vi "SetGetMeasMode - Test.vi"() -> ()   [LabVIEW 2017]
uses:
  AT901 API/TypeDefinitions/ES_MeasMode.ctl
panel:
  out "Command 2":string
  out "Respond 2":string[](array[string])
  out "ES_MeasMode 2":T1
  out "Command":string
  out "Respond":string[](array[string])
  in  "ES_MeasMode":T1
  out "error out":errorcluster
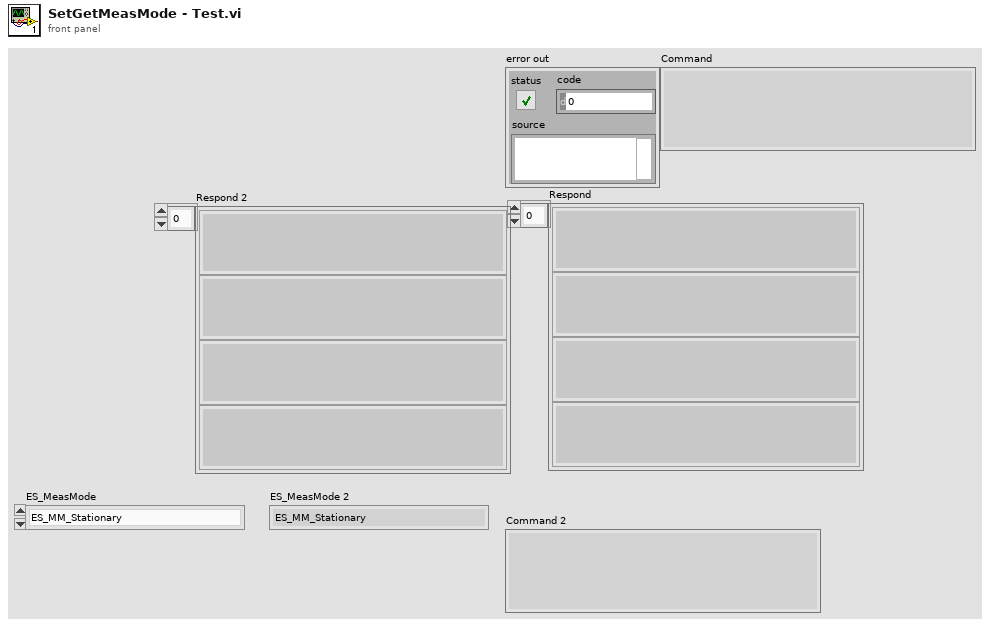
[diagram p1: front panel]
types:
  T1 = typedef "ES_MeasMode.ctl" = enum32{"ES_MM_Stationary", "ES_MM_ContinuousTime", "ES_MM_ContinuousDistance", "ES_MM_Grid", "ES_MM_SphrereCenter", "ES_MM_CircleCenter", "ES_MM_6DStationary", "ES_MM_6DContinuousTime", "ES_MM_6DContinuousDistance", "ES_MM_6DGrid", "ES_MM_6DSphrereCenter", "ES_MM6DCircleCenter"}
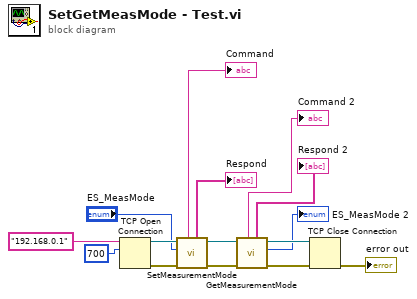
[diagram p0: block diagram]
diagram:
  n1 = TCP Open Connection(address="192.168.0.1", remote port or service name=u16 700) -> (connection ID=w12:refnum<k5>, error out=w7:errorcluster)  [unwired: 3 in]
  n2 = call "SetMeasurementMode.vi"("error in (no error)"=w7, "ES_MeasMode"="ES_MeasMode", "TCP Network Connection in"=w12) -> ("error out"=w8:errorcluster, "TCP Network Connection out"=w11:refnum<k5>, "Respond"=→"Respond":string[], "Command"=→"Command":string)  [unwired: 5 in]
  n3 = call "GetMeasurementMode.vi"("error in (no error)"=w8, "TCP Network Connection in"=w11) -> ("error out"=w9:errorcluster, "ES_MeasMode"=→"ES_MeasMode 2":T1, "TCP Network Connection out"=w10:refnum<k5>, "Respond"=→"Respond 2":string[], "Command"=→"Command 2":string)  [unwired: 5 in]
  n4 = TCP Close Connection(connection ID=w10, error in (no error)=w9) -> (error out=→"error out":errorcluster)  [unwired: 1 in, 1 out]
